vi "Delta_Arrays_Equal_To_Zero.vi"(6 "max difference (0)":i32, 9 "Current Manipulator Position":i32[](array[numeric]), 11 "Next Scan Position":i32[](array[numeric])) -> (2 "At Pos?":bool)   [LabVIEW 2018]
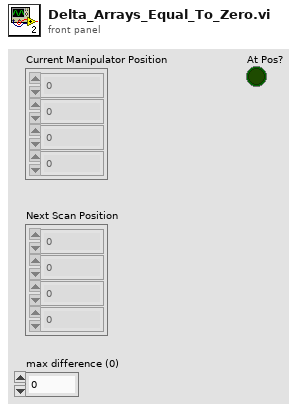
[diagram p1: front panel]
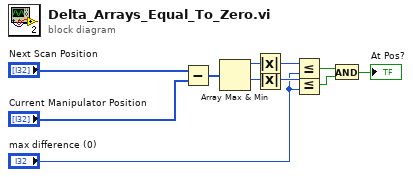
[diagram p0: block diagram]
diagram:
  n1 = Subtract(x="Next Scan Position", y="Current Manipulator Position") -> (x-y=w9:i32[])
  n2 = Array Max & Min(array=w9) -> (max value=w8:i32, min value=w7:i32)  [unwired: 2 out]
  n3 = Absolute Value(x=w8) -> (abs(x)=w5:i32)
  n4 = Absolute Value(x=w7) -> (abs(x)=w4:i32)
  n5 = Less Or Equal?(x=w5, y="max difference (0)") -> (x <= y?=w3:bool)
  n6 = Less Or Equal?(x=w4, y="max difference (0)") -> (x <= y?=w2:bool)
  n7 = And(x=w3, y=w2) -> (x .and. y?=→"At Pos?":bool)
